vi "Client.vi"() -> ()   [LabVIEW 2023]
uses:
  <vilib>/Utility/error.llb/Trim Whitespace One-Sided.vi
  System.Speech
  <vilib>/Utility/file.llb/Read Delimited Spreadsheet (string).vi
  System.Windows.Forms
panel:
  in  "Path":path
  out "Boolean 2":bool
  in  "password 3":string
  in  "Username 2":string
  out "element":string
  out "String":string
  out "Boolean":bool
  out "CorrectPassword":string[](array[string])
  out "Username":string[](array[string])
  out "Numeric":dbl
  out "keep actual volume":dbl
  in  "WindowsMediaPlayer":refnum<k7>(container)
  in  "Tab Control":T1(tab)
  in  "log Button":bool
  out "Gauge":dbl(knob) scale=0.0..260.0
  in  "Welcome Back button":bool
  in  "login Button":bool
  in  "back to welcome back":bool
  out "current time":timestamp format="%<%x>T"
  out "current time 2":timestamp format="%<%I:%M %p>T"
  in  "Password 2":T2
  out "Password":string
  in  "Outer Control":bool
  in  "Inner Control":bool
  in  "Main Menu Log Out":bool
  in  "Radio":bool
  in  "Broswer":bool
  in  "Door Control":bool
  out "current time 22":timestamp format="%<%x>T"
  out "current time 21":timestamp format="%<%I:%M %p>T"
  in  "Door control Back to Main Menu":bool
  in  "Back Left Door":bool
  in  "Back Right Door":bool
  in  "Front Right Door":bool
  in  "Close All Doors":bool
  in  "Lock All Doors":bool
  in  "Front Left Door":bool
  out "current time 4":timestamp format="%<%x>T"
  out "current time 3":timestamp format="%<%I:%M %p>T"
  in  "Window  Child Lock":bool
  in  "Close All Windows":bool
  in  "Close Moonroof":bool
  in  "Trunk 2":bool
  in  "Bonnet 2":bool
  in  "Right Back Window":dbl(knob) scale=0.0..100.0
  in  "Right Front Window":dbl(knob) scale=0.0..100.0
  in  "Left Back Window":dbl(knob) scale=0.0..100.0
  in  "Left Front Window":dbl(knob) scale=0.0..100.0
  in  "Outer Control Back to Main Menu":bool
  in  "High Light Beam":bool
  in  "Low Light Beam":bool
  out "current time 6":timestamp format="%<%x>T"
  out "current time 5":timestamp format="%<%I:%M %p>T"
  in  "Oil Tank":bool
  in  "Siri button":bool
  in  "View 360":bool
  in  "Tempurature":u8(slide) scale=16.0..24.0
  out "Numeric 2":dbl
  out "Ac light":bool
  in  "On/Off Ac":bool
  in  "On/Off fan":bool
  out "Numeric 3":dbl
  in  "Call":bool
  in  "Password 4":T3
  out "Password 3":string
  in  "Inner Control Back to Main Menu":bool
  out "fan light":bool
  in  "Fan Speed":u8(slide) scale=1.0..5.0
  in  "Double Signal":bool
  out "current time 24":timestamp format="%<%x>T"
  out "current time 23":timestamp format="%<%I:%M %p>T"
  out "Display channel":string
  in  "ONOFF":bool
  in  "Radio Back to main menu":bool
  in  "Unmute":bool
  in  "109.90":bool
  in  "98.80":bool
  in  "105.90":bool
  in  "92.90":bool
  in  "102.90":bool
  in  "91.10":bool
  in  "101.90":bool
  in  "89.90":bool
  in  "Volume slider":u8(slide) scale=0.0..100.0
  out "current time 10":timestamp format="%<%x>T"
  out "current time 9":timestamp format="%<%I:%M %p>T"
  in  "Miscrsoft button":bool
  in  "Netflix Button":bool
  in  "Enter Url":string
  in  "Browser Back to Main Menu":bool
  in  "Gmail button":bool
  in  "Facebook button":bool
  out "current time 8":timestamp format="%<%x>T"
  out "current time 7":timestamp format="%<%I:%M %p>T"
  in  "Search Button":bool
  in  "Google Button":bool
  in  "Display Browser Back to main menu":bool
  out "current time 12":timestamp format="%<%x>T"
  out "current time 11":timestamp format="%<%I:%M %p>T"
  in  "WebBrowser":refnum<k24>(container)
  in  "360view back to main menu":bool
  out "current time 16":timestamp format="%<%x>T"
  out "current time 15":timestamp format="%<%I:%M %p>T"
  # "Welcome Back"
  # "PROTON AZ5"
  # "Enter Passcode"
  # "Main Menu"
  # "Door\nControl"
  # "Outer \nControl"
  # "Phone Call"
  # "Inner \nControl"
  # "Radio"
  # "Browser"
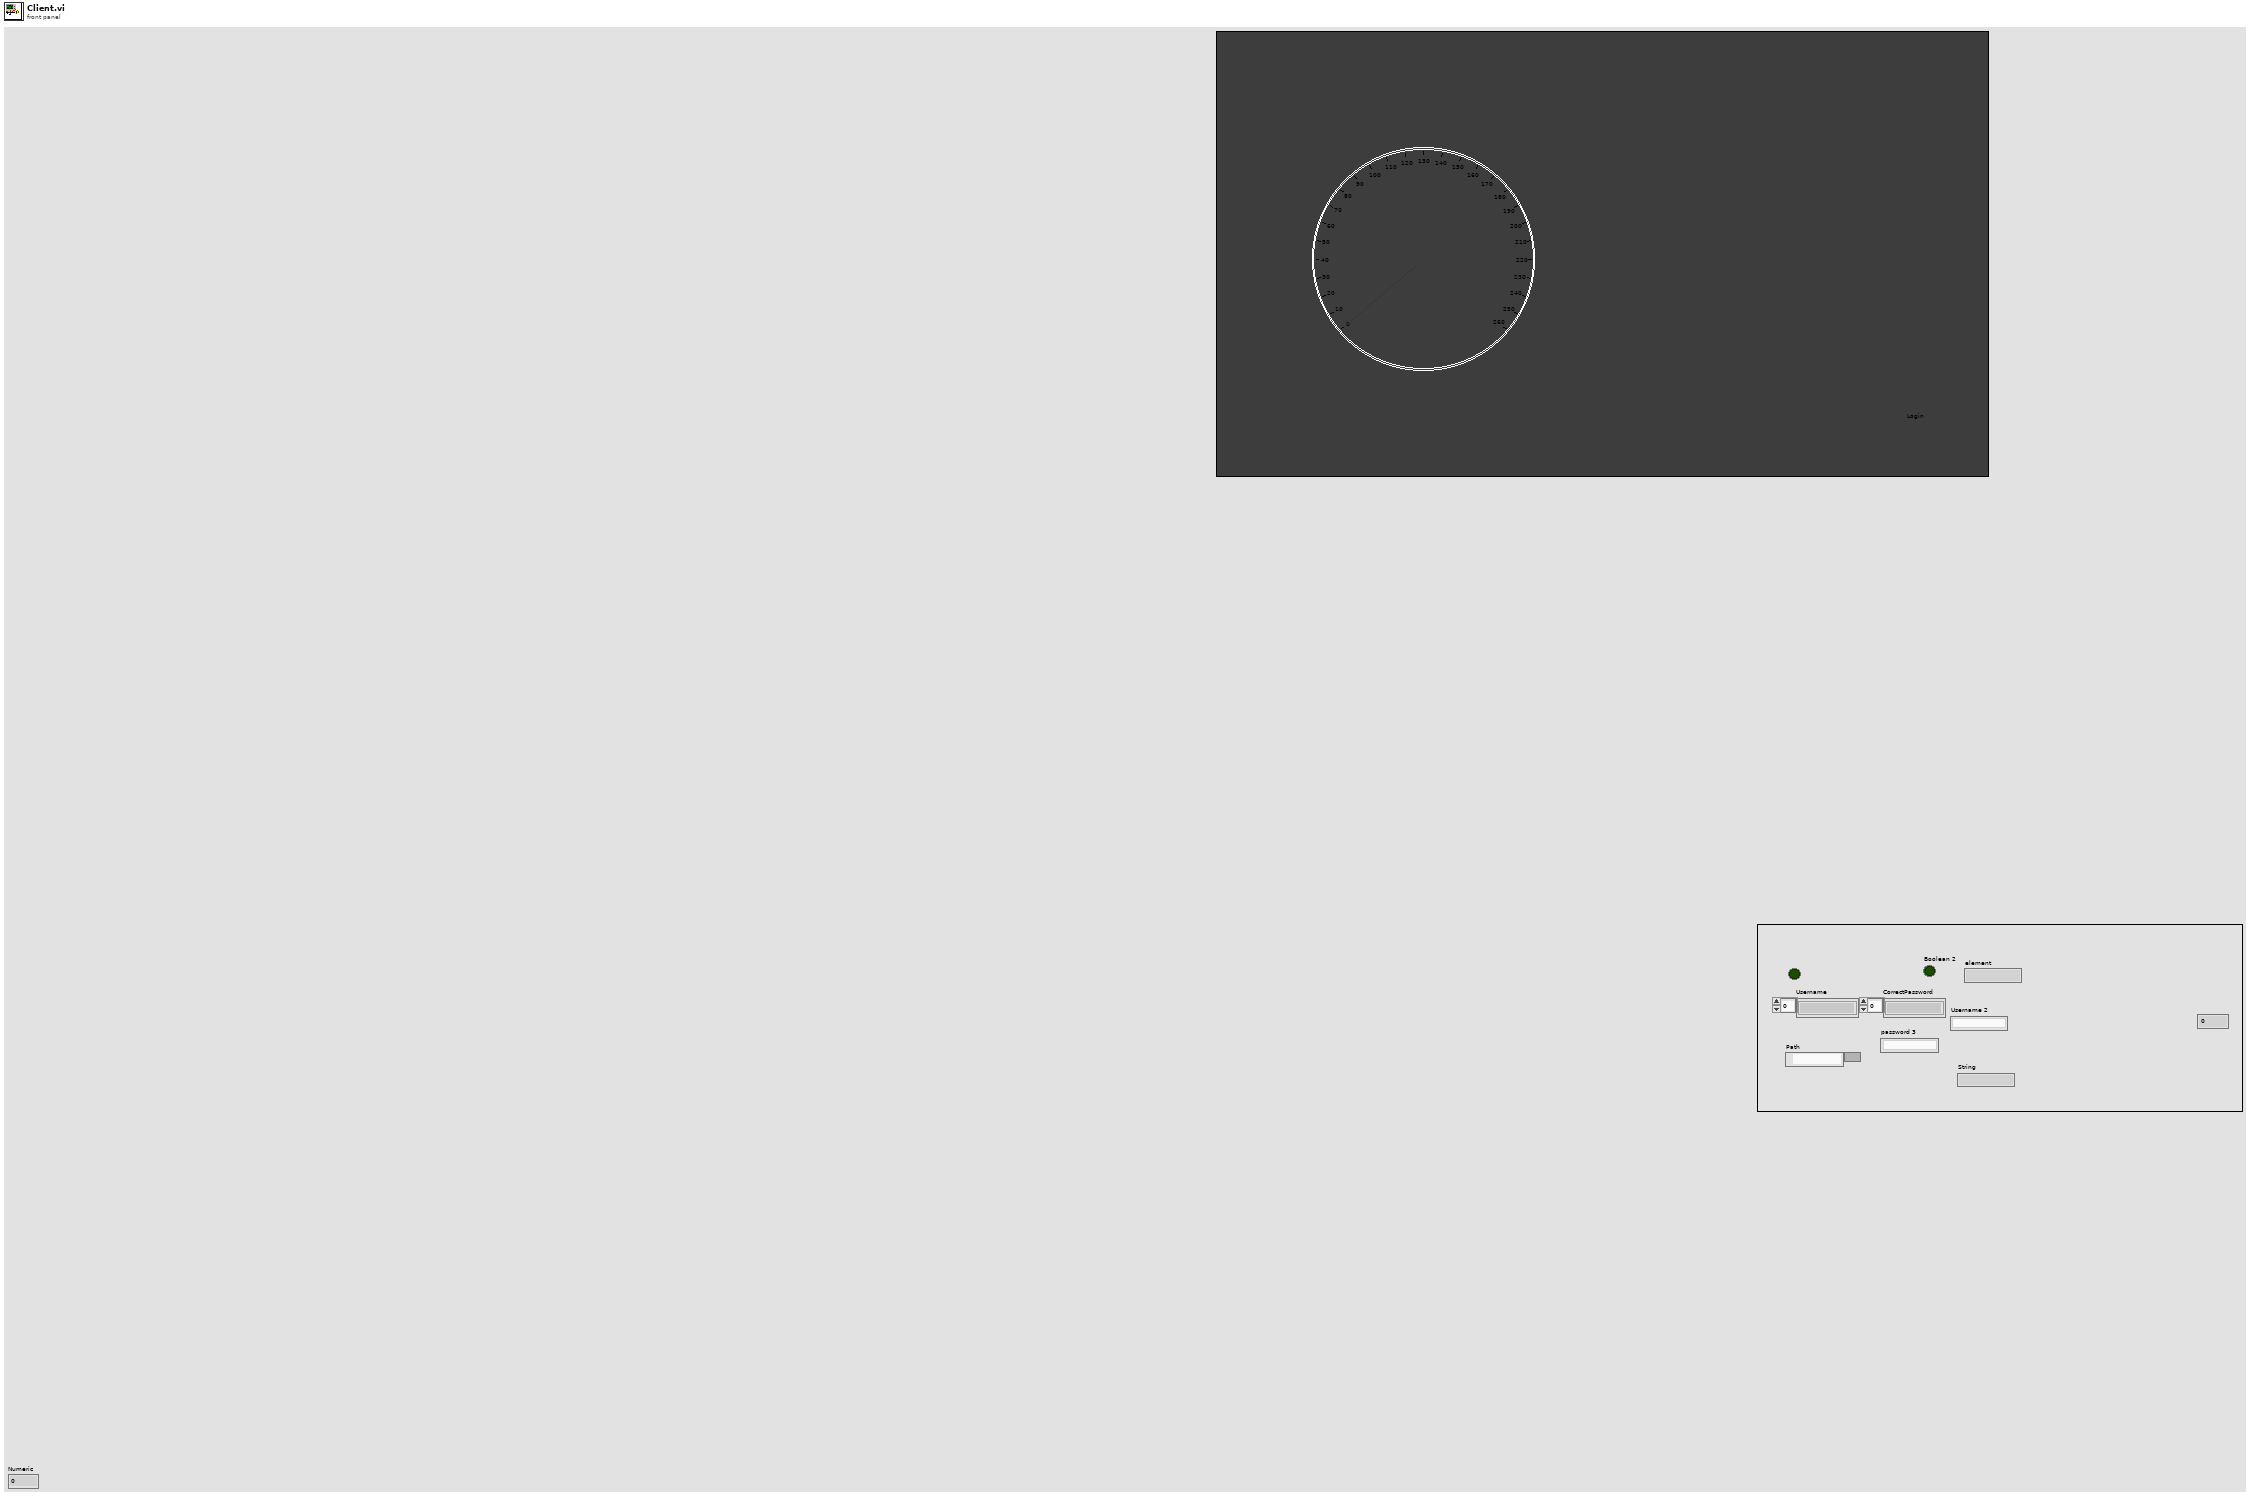
[diagram p1: front panel]
types:
  T1 = enum32{"Meter", "Login Page", "Main Menu", "Door Control", "Outer Control", "Inner Control", "Radio", "Browser", "Display Browser", "360view"}
  T2 = cluster{"1":bool, "2":bool, "4":bool, "5":bool, "6":bool, "7":bool, "8":bool, "9":bool, "0":bool, "3":bool, "Refresh Button":bool}
  T3 = cluster{"Call N1":bool, "Call N2":bool, "Call N3":bool, "Call N4":bool, "Call N5":bool, "Call N6":bool, "Call N7":bool, "Call N8":bool, "Call N9":bool, "Call N0":bool, "Clear":bool}
  T4 = enum32{"Login Page", "Menu Page", "Door Page", "Light Page", "Window Page", "Radio Page", "Browsing Page", "Advanced Setting", "Profile Page"}
  T5 = enum8{"Enabled", "Disabled", "Disabled and Grayed Out"}
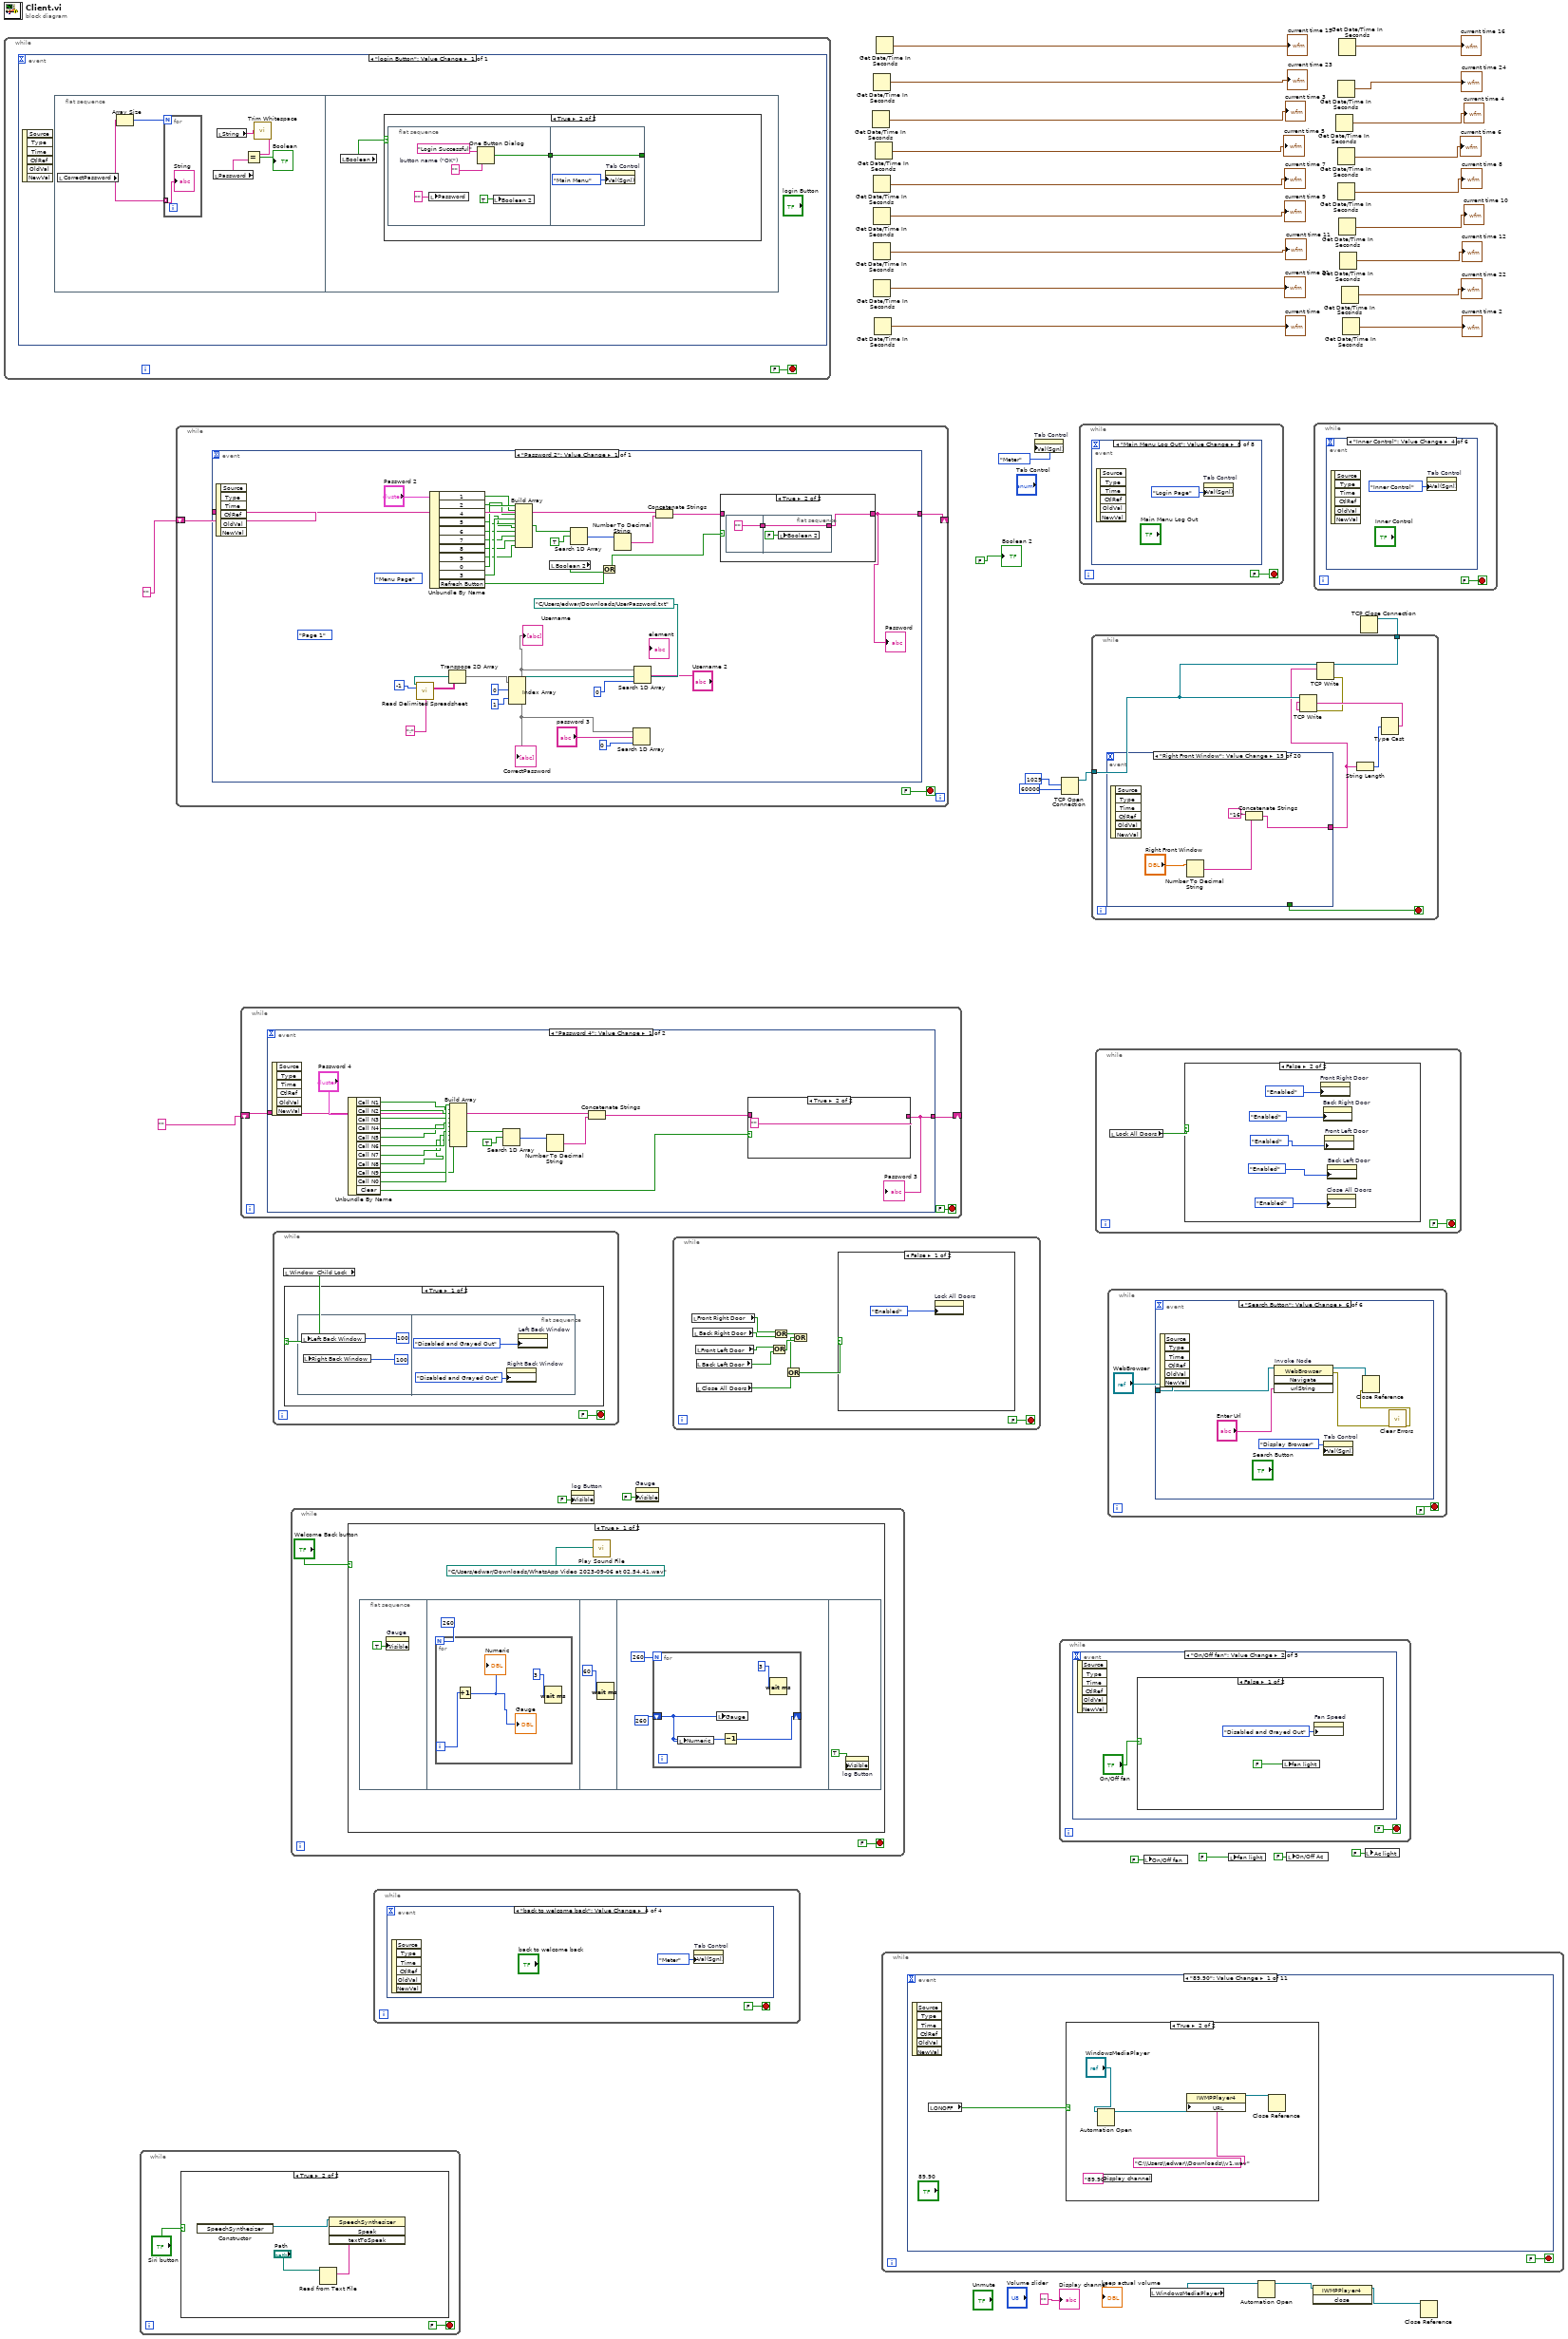
[diagram p0: block diagram]
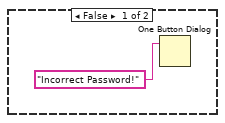
[diagram p3: hidden frame]
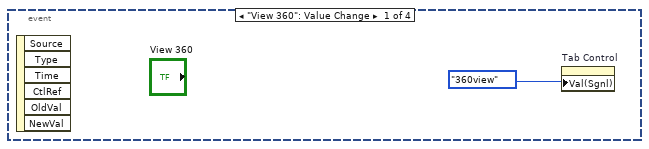
[diagram p4: hidden frame]
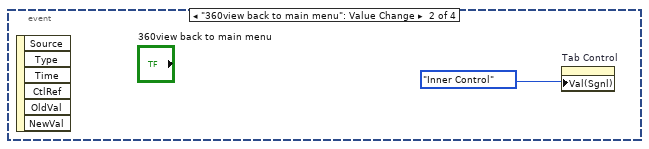
[diagram p5: hidden frame]
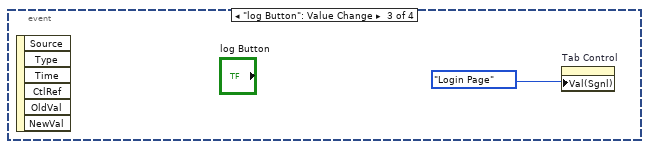
[diagram p6: hidden frame]
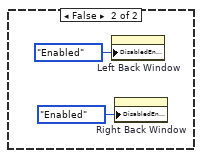
[diagram p8: hidden frame]
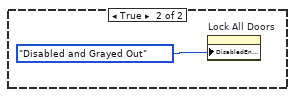
[diagram p9: hidden frame]
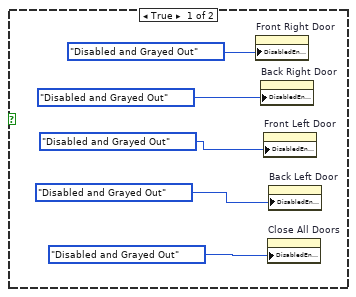
[diagram p10: hidden frame]
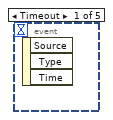
[diagram p11: hidden frame]
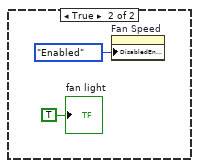
[diagram p12: hidden frame]
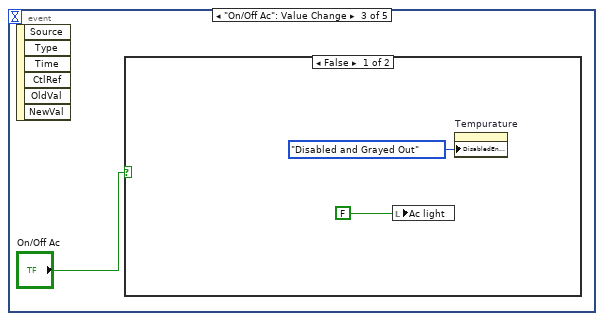
[diagram p13: hidden frame]
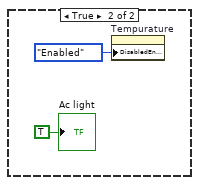
[diagram p14: hidden frame]
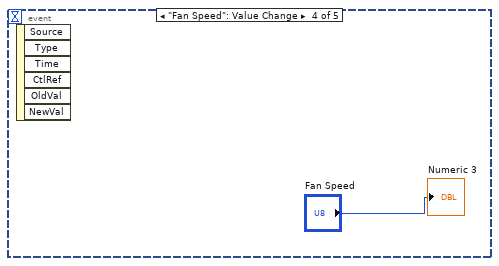
[diagram p15: hidden frame]
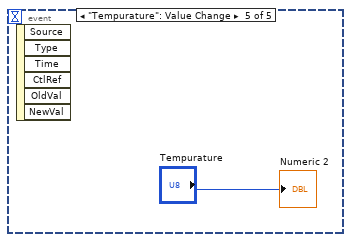
[diagram p16: hidden frame]
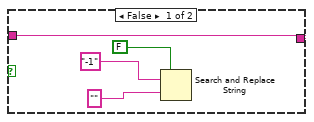
[diagram p17: hidden frame]
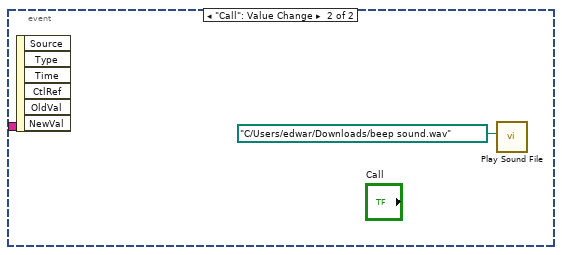
[diagram p18: hidden frame]
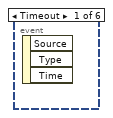
[diagram p19: hidden frame]
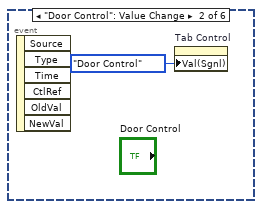
[diagram p20: hidden frame]
diagram:
  n1 = while {
    stop <- FALSE stop-if-true
    n2 = event shown="[0] \"login Button\": Value Change" {
      selector: _ -> [_]
      dyn-events: _ -> [_]
      timeout: _ -> [_]
      event "login Button": Value Change {
        n3 = event-data() -> ()  [unwired: 1 in, 6 out]
        n4 = flat-sequence {
          frame #0 {
            n5 = local read "CorrectPassword"() -> (w42:string[])
            n6 = Array Size(array=w42) -> (size(s)=w43:i32)
            n7 = for {
              N: w43 -> [_]
              tunnel: w42 -> [w44] mode=indexing
              "String" <- w44
            }
            n8 = local read "Password"() -> (w38:string)
            n9 = local read "String"() -> (w40:string)
            n10 = call <vilib>:"Trim Whitespace.vi"("string"=w40) -> ("trimmed string"=w39:string)  [unwired: 1 in]
            n11 = Equal?(x=w39, y=w38) -> (x = y?=→"Boolean":bool)
          }
          frame #1 {
            n12 = local read "Boolean"() -> (w45:bool)
            n13 = case shown="True" w45 {
              frame False {
                n14 = One Button Dialog(message="Incorrect Password!") -> ()  [unwired: 1 in, 1 out]
              }
              frame True {
                n15 = flat-sequence {
                  tunnel: [w48] -> w47
                  tunnel: [w53] -> _
                  tunnel: w47 -> [w53]
                  frame #0 {
                    w51 = ""  # button name ("OK")
                    n16 = local write "Password"("" ("Passsword")) -> ()
                    n17 = One Button Dialog(message="Login Successful", button name ("OK")=w51) -> (true=w48:bool)
                    n18 = local write "Boolean 2"(TRUE ("Boolean 2")) -> ()
                  }
                  frame #1 {
                    n19 = property on="Tab Control" class="TabCtl (strict)"("Val(Sgnl)"=T1."Main Menu" ("Value (Signaling)")) -> ()  [unwired: 2 in, 2 out]
                  }
                }
              }
            }
          }
        }
      }
    }
  }
  n20 = while {
    stop <- FALSE stop-if-true
    n21 = case shown="True" "Siri button" {
      frame False {
      }
      frame True {
        n22 = constructor class="SpeechSynthesizer"() -> (reference out=w59:refnum<k24>)  [unwired: 3 in, 2 out]
        n23 = Read from Text File(file (use dialog)="Path") -> (text=w57:string)  [unwired: 3 in, 3 out]
        n24 = invoke class="SpeechSynthesizer" method="Speak"(reference=w59, "textToSpeak"=w57) -> ()  [unwired: 2 in, 4 out]
      }
    }
  }
  n25 = while {
    shift-right: [w60] -> _
    shift-left: "" -> [w61]
    stop <- FALSE stop-if-true
    n26 = event shown="[0] \"Password 2\": Value Change" {
      selector: _ -> [_]
      dyn-events: _ -> [_]
      timeout: _ -> [_]
      tunnel: w61 -> [w92]
      tunnel: [w68] -> w60
      event "Password 2": Value Change {
        (unwired) T4."Menu Page" ("Value (Signaling)")
        (unwired) enum32{"Page 1", "Page 2"}."Page 1" ("Tab Control 12")
        n27 = event-data() -> ()  [unwired: 1 in, 6 out]
        n28 = call-poly <vilib>:"Read Delimited Spreadsheet.vi"("file path (dialog if empty)"=path "C:/Users/edwar/Downloads/UserPassword.txt", "number of rows (all:-1)"=-1, "delimiter (\\t)"=":" ("delimiter (\\t)")) -> ("all rows"=w79:string[][])  [unwired: 7 in, 5 out]
        n29 = Unbundle By Name "Unbundle By Name"("Password 2") -> ("1"=w90:bool, "2"=w89:bool, "4"=w87:bool, "5"=w86:bool, "6"=w85:bool, "7"=w84:bool, "8"=w83:bool, "9"=w82:bool, "0"=w91:bool, "3"=w88:bool, "Refresh Button"=w65:bool)
        n30 = Transpose 2D Array(2D array=w79) -> (transposed array=w78:string[][])
        n31 = Index Array(array=w78, index (row) #1=0 ("index (row)"), index (row) #2=1 ("index (row)")) -> (element #1=w70:string[], element #2=w69:string[])  [unwired: 2 in]
        "Username" <- w70
        "CorrectPassword" <- w69
        n32 = Build Array "Build Array"(w91, w90, w89, w88, w87, w86, w85, w84, w83, w82) -> (w95:bool[])
        n33 = local read "Boolean 2"() -> (w63:bool)
        n34 = Search 1D Array(1D array=w95, element=TRUE) -> (index of element=w94:i32)  [unwired: 1 in]
        n35 = Or(x=w65, y=w63) -> (x .or. y?=w64:bool)
        n36 = Number To Decimal String(number=w94) -> (decimal integer string=w93:string)  [unwired: 1 in]
        n37 = Search 1D Array(1D array=w69, element="password 3", start index (0)=0) -> ()  [unwired: 1 out]
        n38 = Search 1D Array(1D array=w70, element="Username 2", start index (0)=0) -> ()  [unwired: 1 out]
        n39 = Concatenate Strings "Concatenate Strings"(w92, w93) -> (w80:string)
        n40 = case shown="True" w64 {
          tunnel: w80 -> [w97 _]
          tunnel: [w97 w102] -> w68
          frame False {
            n41 = Search and Replace String(replace all?=FALSE ("replace all? (F)"), input string="", search string="-1") -> ()  [unwired: 5 in, 4 out]
          }
          frame True {
            n42 = flat-sequence {
              tunnel: [""] -> w101
              tunnel: [w105] -> w102
              tunnel: w101 -> [w105]
              frame #0 {
              }
              frame #1 {
                n43 = local write "Boolean 2"(FALSE ("Boolean 2")) -> ()
              }
            }
          }
        }
        "Password" <- w68
      }
    }
  }
  n44 = while {
    shift-right: [w108] -> _
    shift-left: "" -> [w107]
    stop <- FALSE stop-if-true
    n45 = event shown="[0] \"Password 4\": Value Change" {
      selector: _ -> [_ _]
      dyn-events: _ -> [_ _]
      timeout: _ -> [_ _]
      tunnel: [w110 _] -> w108
      tunnel: w107 -> [w111 _]
      event "Password 4": Value Change {
        n46 = event-data() -> ()  [unwired: 1 in, 6 out]
        n47 = Unbundle By Name("Password 4") -> ("Call N1"=w125:bool, "Call N2"=w124:bool, "Call N3"=w123:bool, "Call N4"=w122:bool, "Call N5"=w121:bool, "Call N6"=w120:bool, "Call N7"=w119:bool, "Call N8"=w118:bool, "Call N9"=w117:bool, "Call N0"=w126:bool, "Clear"=w109:bool)
        n48 = Build Array "Build Array"(w126, w125, w124, w123, w122, w121, w120, w119, w118, w117) -> (w112:bool[])
        n49 = Search 1D Array(1D array=w112, element=TRUE) -> (index of element=w116:i32)  [unwired: 1 in]
        n50 = Number To Decimal String(number=w116) -> (decimal integer string=w115:string)  [unwired: 1 in]
        n51 = Concatenate Strings "Concatenate Strings"(w111, w115) -> (w113:string)
        n52 = case shown="True" w109 {
          tunnel: w113 -> [w128 _]
          tunnel: [w128 ""] -> w110
          frame False {
            n53 = Search and Replace String(replace all?=FALSE ("replace all? (F)"), input string="", search string="-1") -> ()  [unwired: 5 in, 4 out]
          }
          frame True {
          }
        }
        "Password 3" <- w110
      }
      event "Call": Value Change {
        n54 = event-data() -> ()  [unwired: 1 in, 6 out]
        n55 = call <vilib>:"Play Sound File.vi"("path"=path "C:/Users/edwar/Downloads/beep sound.wav") -> ()  [unwired: 9 in, 2 out]
      }
    }
  }
  n56 = while {
    stop <- FALSE stop-if-true
    n57 = local read "Window  Child Lock"() -> (w134:bool)
    n58 = case shown="True" w134 {
      frame True {
        n59 = flat-sequence {
          frame #0 {
            n60 = local write "Left Back Window"(100) -> ()
            n61 = local write "Right Back Window"(100) -> ()
          }
          frame #1 {
            n62 = property on="Right Back Window" class="Knob (strict)"("DisabledEnum"=T5."Disabled and Grayed Out" ("Disabled")) -> ()  [unwired: 2 in, 2 out]
            n63 = property on="Left Back Window" class="Knob (strict)"("DisabledEnum"=T5."Disabled and Grayed Out" ("Disabled")) -> ()  [unwired: 2 in, 2 out]
          }
        }
      }
      frame False {
        n64 = property on="Left Back Window" class="Knob (strict)"("DisabledEnum"=T5."Enabled" ("Disabled")) -> ()  [unwired: 2 in, 2 out]
        n65 = property on="Right Back Window" class="Knob (strict)"("DisabledEnum"=T5."Enabled" ("Disabled")) -> ()  [unwired: 2 in, 2 out]
      }
    }
  }
  n66 = while {
    stop <- FALSE stop-if-true
    n67 = case shown="True" "Welcome Back button" {
      frame True {
        n68 = flat-sequence {
          frame #0 {
            n69 = property on="Gauge" class="Knob (strict)"("Visible"=TRUE) -> ()  [unwired: 2 in, 2 out]
          }
          frame #1 {
            n70 = for {
              N: 260 -> [_]
              i -> [w149]
              n71 = Increment(x=w149) -> (x+1=→"Numeric" →"Gauge":i32)
              n72 = Wait (ms)(milliseconds to wait=u32 3) -> ()  [unwired: 1 out]
            }
          }
          frame #2 {
            n73 = Wait (ms)(milliseconds to wait=u32 60) -> ()  [unwired: 1 out]
          }
          frame #3 {
            n74 = for {
              N: 260 -> [_]
              shift-right: [w153] -> _
              shift-left: 260 -> [w154]
              n75 = local write "Numeric"(w154) -> ()
              n76 = local write "Gauge"(w154) -> ()
              n77 = Decrement(x=w154) -> (x-1=w153:i32)
              n78 = Wait (ms)(milliseconds to wait=u32 3) -> ()  [unwired: 1 out]
            }
          }
          frame #4 {
            n79 = property on="log Button" class="Bool"("Visible"=TRUE) -> ()  [unwired: 2 in, 2 out]
          }
        }
        n80 = call <vilib>:"Play Sound File.vi"("path"=path "C:/Users/edwar/Downloads/WhatsApp Video 2023-09-06 at 02.54.41.wav") -> ()  [unwired: 9 in, 2 out]
      }
      frame False {
      }
    }
  }
  n81 = while {
    stop <- FALSE stop-if-true
    n82 = event shown="[3] \"back to welcome back\": Value Change" {
      selector: _ -> [_ _ _ _]
      dyn-events: _ -> [_ _ _ _]
      timeout: _ -> [_ _ _ _]
      event "View 360": Value Change {
        n83 = event-data() -> ()  [unwired: 1 in, 6 out]
        n84 = property on="Tab Control" class="TabCtl (strict)"("Val(Sgnl)"=T1."360view" ("Value (Signaling)")) -> ()  [unwired: 2 in, 2 out]
      }
      event "360view back to main menu": Value Change {
        n85 = event-data() -> ()  [unwired: 1 in, 6 out]
        n86 = property on="Tab Control" class="TabCtl (strict)"("Val(Sgnl)"=T1."Inner Control" ("Value (Signaling)")) -> ()  [unwired: 2 in, 2 out]
      }
      event "log Button": Value Change {
        n87 = event-data() -> ()  [unwired: 1 in, 6 out]
        n88 = property on="Tab Control" class="TabCtl (strict)"("Val(Sgnl)"=T1."Login Page" ("Value (Signaling)")) -> ()  [unwired: 2 in, 2 out]
      }
      event "back to welcome back": Value Change {
        n89 = event-data() -> ()  [unwired: 1 in, 6 out]
        n90 = property on="Tab Control" class="TabCtl (strict)"("Val(Sgnl)"=T1."Meter" ("Value (Signaling)")) -> ()  [unwired: 2 in, 2 out]
      }
    }
  }
  n91 = property on="log Button" class="Bool"("Visible"=FALSE) -> ()  [unwired: 2 in, 2 out]
  n92 = property on="Gauge" class="Knob (strict)"("Visible"=FALSE) -> ()  [unwired: 2 in, 2 out]
  n93 = while {
    stop <- FALSE stop-if-true
    n94 = local read "Front Right Door"() -> (w171:bool)
    n95 = local read "Back Right Door"() -> (w168:bool)
    n96 = local read "Front Left Door"() -> (w167:bool)
    n97 = local read "Back Left Door"() -> (w166:bool)
    n98 = local read "Close All Doors"() -> (w164:bool)
    n99 = Or(x=w167, y=w166) -> (x .or. y?=w169:bool)
    n100 = Or(x=w171, y=w168) -> (x .or. y?=w170:bool)
    n101 = Or(x=w170, y=w169) -> (x .or. y?=w163:bool)
    n102 = Or(x=w163, y=w164) -> (x .or. y?=w162:bool)
    n103 = case shown="False" w162 {
      frame False {
        n104 = property on="Lock All Doors" class="Bool (strict)"("DisabledEnum"=T5."Enabled" ("Disabled")) -> ()  [unwired: 2 in, 2 out]
      }
      frame True {
        n105 = property on="Lock All Doors" class="Bool (strict)"("DisabledEnum"=T5."Disabled and Grayed Out" ("Disabled")) -> ()  [unwired: 2 in, 2 out]
      }
    }
  }
  n106 = Get Date/Time In Seconds() -> (seconds since 1Jan1904=→"current time 3":timestamp)
  n107 = Get Date/Time In Seconds() -> (seconds since 1Jan1904=→"current time 7":timestamp)
  n108 = Get Date/Time In Seconds() -> (seconds since 1Jan1904=→"current time 9":timestamp)
  n109 = Get Date/Time In Seconds() -> (seconds since 1Jan1904=→"current time 11":timestamp)
  n110 = Get Date/Time In Seconds() -> (seconds since 1Jan1904=→"current time 23":timestamp)
  n111 = Get Date/Time In Seconds() -> (seconds since 1Jan1904=→"current time 21":timestamp)
  n112 = Get Date/Time In Seconds() -> (seconds since 1Jan1904=→"current time":timestamp)
  n113 = Get Date/Time In Seconds() -> (seconds since 1Jan1904=→"current time 5":timestamp)
  n114 = Get Date/Time In Seconds() -> (seconds since 1Jan1904=→"current time 15":timestamp)
  n115 = while {
    stop <- FALSE stop-if-true
    n116 = event shown="[0] \"89.90\": Value Change" {
      selector: _ -> [_ _ _ _ _ _ _ _ _ _ _]
      dyn-events: _ -> [_ _ _ _ _ _ _ _ _ _ _]
      timeout: _ -> [_ _ _ _ _ _ _ _ _ _ _]
      event "89.90": Value Change {
        n117 = event-data() -> ()  [unwired: 1 in, 6 out]
        n118 = local read "ONOFF"() -> (w175:bool)
        n119 = case shown="True" w175 {
          frame False {
            n120 = One Button Dialog(message="Please turn on the radio", button name ("OK")="") -> ()  [unwired: 1 out]
          }
          frame True {
            n121 = local write "Display channel"("89.90" ("String")) -> ()
            n122 = Automation Open(Automation Refnum="WindowsMediaPlayer") -> (Automation Refnum=w180:refnum<k7>)  [unwired: 3 in, 1 out]
            n123 = property class="IWMPPlayer4"(reference=w180, "URL"="C:\\Users\\edwar\\Downloads\\v1.wav") -> (reference out=w182:refnum<k7>)  [unwired: 1 in, 1 out]
            n124 = Close Reference(reference=w182) -> ()  [unwired: 1 in, 1 out]
          }
        }
      }
      event "91.10": Value Change {
        n125 = event-data() -> ()  [unwired: 1 in, 6 out]
        n126 = local read "ONOFF"() -> (w183:bool)
        n127 = case shown="True" w183 {
          frame False {
            n128 = One Button Dialog(message="Please turn on the radio", button name ("OK")="") -> ()  [unwired: 1 out]
          }
          frame True {
            n129 = local read "WindowsMediaPlayer"() -> (w186:refnum<k7>)
            n130 = local write "Display channel"("91.90" ("String")) -> ()
            n131 = Automation Open(Automation Refnum=w186) -> (Automation Refnum=w189:refnum<k7>)  [unwired: 3 in, 1 out]
            n132 = property class="IWMPPlayer4"(reference=w189, "URL"="C:\\Users\\edwar\\Downloads\\v2.wav") -> (reference out=w190:refnum<k7>)  [unwired: 1 in, 1 out]
            n133 = Close Reference(reference=w190) -> ()  [unwired: 1 in, 1 out]
          }
        }
      }
      event "92.90": Value Change {
        n134 = event-data() -> ()  [unwired: 1 in, 6 out]
        n135 = local read "ONOFF"() -> (w191:bool)
        n136 = case shown="True" w191 {
          frame False {
            n137 = One Button Dialog(message="Please turn on the radio", button name ("OK")="") -> ()  [unwired: 1 out]
          }
          frame True {
            n138 = local read "WindowsMediaPlayer"() -> (w194:refnum<k7>)
            n139 = local write "Display channel"("92.90" ("String")) -> ()
            n140 = Automation Open(Automation Refnum=w194) -> (Automation Refnum=w197:refnum<k7>)  [unwired: 3 in, 1 out]
            n141 = property class="IWMPPlayer4"(reference=w197, "URL"="C:\\Users\\edwar\\Downloads\\v3.wav") -> (reference out=w198:refnum<k7>)  [unwired: 1 in, 1 out]
            n142 = Close Reference(reference=w198) -> ()  [unwired: 1 in, 1 out]
          }
        }
      }
      event "98.80": Value Change {
        n143 = event-data() -> ()  [unwired: 1 in, 6 out]
        n144 = local read "ONOFF"() -> (w199:bool)
        n145 = case shown="True" w199 {
          frame False {
            n146 = One Button Dialog(message="Please turn on the radio", button name ("OK")="") -> ()  [unwired: 1 out]
          }
          frame True {
            n147 = local read "WindowsMediaPlayer"() -> (w202:refnum<k7>)
            n148 = local write "Display channel"("98.80" ("String")) -> ()
            n149 = Automation Open(Automation Refnum=w202) -> (Automation Refnum=w205:refnum<k7>)  [unwired: 3 in, 1 out]
            n150 = property class="IWMPPlayer4"(reference=w205, "URL"="C:\\Users\\edwar\\Downloads\\v4.wav") -> (reference out=w206:refnum<k7>)  [unwired: 1 in, 1 out]
            n151 = Close Reference(reference=w206) -> ()  [unwired: 1 in, 1 out]
          }
        }
      }
      event "101.90": Value Change {
        n152 = event-data() -> ()  [unwired: 1 in, 6 out]
        n153 = local read "ONOFF"() -> (w207:bool)
        n154 = case shown="True" w207 {
          frame False {
            n155 = One Button Dialog(message="Please turn on the radio", button name ("OK")="") -> ()  [unwired: 1 out]
          }
          frame True {
            n156 = local read "WindowsMediaPlayer"() -> (w210:refnum<k7>)
            n157 = local write "Display channel"("101.90" ("String")) -> ()
            n158 = Automation Open(Automation Refnum=w210) -> (Automation Refnum=w213:refnum<k7>)  [unwired: 3 in, 1 out]
            n159 = property class="IWMPPlayer4"(reference=w213, "URL"="C:\\Users\\edwar\\Downloads\\v5.wav") -> (reference out=w214:refnum<k7>)  [unwired: 1 in, 1 out]
            n160 = Close Reference(reference=w214) -> ()  [unwired: 1 in, 1 out]
          }
        }
      }
      event "102.90": Value Change {
        n161 = event-data() -> ()  [unwired: 1 in, 6 out]
        n162 = local read "ONOFF"() -> (w215:bool)
        n163 = case shown="True" w215 {
          frame False {
            n164 = One Button Dialog(message="Please turn on the radio", button name ("OK")="") -> ()  [unwired: 1 out]
          }
          frame True {
            n165 = local read "WindowsMediaPlayer"() -> (w218:refnum<k7>)
            n166 = local write "Display channel"("102.90" ("String")) -> ()
            n167 = Automation Open(Automation Refnum=w218) -> (Automation Refnum=w221:refnum<k7>)  [unwired: 3 in, 1 out]
            n168 = property class="IWMPPlayer4"(reference=w221, "URL"="C:\\Users\\edwar\\Downloads\\v6.wav") -> (reference out=w222:refnum<k7>)  [unwired: 1 in, 1 out]
            n169 = Close Reference(reference=w222) -> ()  [unwired: 1 in, 1 out]
          }
        }
      }
      event "105.90": Value Change {
        n170 = event-data() -> ()  [unwired: 1 in, 6 out]
        n171 = local read "ONOFF"() -> (w223:bool)
        n172 = case shown="True" w223 {
          frame False {
            n173 = One Button Dialog(message="Please turn on the radio", button name ("OK")="") -> ()  [unwired: 1 out]
          }
          frame True {
            n174 = local read "WindowsMediaPlayer"() -> (w226:refnum<k7>)
            n175 = local write "Display channel"("105.90" ("String")) -> ()
            n176 = Automation Open(Automation Refnum=w226) -> (Automation Refnum=w229:refnum<k7>)  [unwired: 3 in, 1 out]
            n177 = property class="IWMPPlayer4"(reference=w229, "URL"="C:\\Users\\edwar\\Downloads\\v7.wav") -> (reference out=w230:refnum<k7>)  [unwired: 1 in, 1 out]
            n178 = Close Reference(reference=w230) -> ()  [unwired: 1 in, 1 out]
          }
        }
      }
      event "109.90": Value Change {
        n179 = event-data() -> ()  [unwired: 1 in, 6 out]
        n180 = local read "ONOFF"() -> (w231:bool)
        n181 = case shown="True" w231 {
          frame False {
            n182 = One Button Dialog(message="Please turn on the radio", button name ("OK")="") -> ()  [unwired: 1 out]
          }
          frame True {
            n183 = local read "WindowsMediaPlayer"() -> (w234:refnum<k7>)
            n184 = local write "Display channel"("109.90" ("String")) -> ()
            n185 = Automation Open(Automation Refnum=w234) -> (Automation Refnum=w237:refnum<k7>)  [unwired: 3 in, 1 out]
            n186 = property class="IWMPPlayer4"(reference=w237, "URL"="C:\\Users\\edwar\\Downloads\\v8.wav") -> (reference out=w238:refnum<k7>)  [unwired: 1 in, 1 out]
            n187 = Close Reference(reference=w238) -> ()  [unwired: 1 in, 1 out]
          }
        }
      }
      event "Unmute": Value Change {
        n188 = event-data() -> ()  [unwired: 1 in, 6 out]
        n189 = local read "Unmute"() -> (w239:bool)
        n190 = case shown="True" w239 {
          frame True {
            n191 = flat-sequence {
              frame #0 {
                n192 = local read "Volume slider"() -> (w240:u8)
                n193 = local write "keep actual volume"(w240) -> ()
              }
              frame #1 {
                n194 = local write "Volume slider"(u8 0 ("Volume slider")) -> ()
              }
              frame #2 {
                n195 = local read "WindowsMediaPlayer"() -> (w246:refnum<k7>)
                n196 = Automation Open(Automation Refnum=w246) -> (Automation Refnum=w245:refnum<k7>)  [unwired: 3 in, 1 out]
                n197 = property class="IWMPPlayer4"(reference=w245) -> ("settings"=w243:refnum<k7>)  [unwired: 1 in, 2 out]
                n198 = local read "Volume slider"() -> (w242:u8)
                n199 = property class="IWMPSettings"(reference=w243, "volume"=w242) -> (reference out=w244:refnum<k7>)  [unwired: 1 in, 1 out]
                n200 = Close Reference(reference=w244) -> ()  [unwired: 1 in, 1 out]
              }
            }
          }
          frame False {
            n201 = flat-sequence {
              frame #0 {
                n202 = local read "keep actual volume"() -> (w247:dbl)
                n203 = local write "Volume slider"(w247) -> ()
              }
              frame #1 {
                n204 = local read "WindowsMediaPlayer"() -> (w251:refnum<k7>)
                n205 = Automation Open(Automation Refnum=w251) -> (Automation Refnum=w250:refnum<k7>)  [unwired: 3 in, 1 out]
                n206 = property class="IWMPPlayer4"(reference=w250) -> ("settings"=w248:refnum<k7>)  [unwired: 1 in, 2 out]
                n207 = local read "Volume slider"() -> (w252:u8)
                n208 = property class="IWMPSettings"(reference=w248, "volume"=w252) -> (reference out=w249:refnum<k7>)  [unwired: 1 in, 1 out]
                n209 = Close Reference(reference=w249) -> ()  [unwired: 1 in, 1 out]
              }
            }
          }
        }
      }
      event "Volume slider": Value Change {
        n210 = event-data() -> ()  [unwired: 1 in, 6 out]
        n211 = local read "WindowsMediaPlayer"() -> (w254:refnum<k7>)
        n212 = Automation Open(Automation Refnum=w254) -> (Automation Refnum=w255:refnum<k7>)  [unwired: 3 in, 1 out]
        n213 = property class="IWMPPlayer4"(reference=w255) -> ("settings"=w257:refnum<k7>)  [unwired: 1 in, 2 out]
        n214 = local read "Volume slider"() -> (w253:u8)
        n215 = property class="IWMPSettings"(reference=w257, "volume"=w253) -> (reference out=w256:refnum<k7>)  [unwired: 1 in, 1 out]
        n216 = Close Reference(reference=w256) -> ()  [unwired: 1 in, 1 out]
      }
      event "ONOFF": Value Change {
        n217 = event-data() -> ()  [unwired: 1 in, 6 out]
        n218 = case shown="True" "ONOFF" {
          frame False {
            n219 = local read "WindowsMediaPlayer"() -> (w260:refnum<k7>)
            n220 = local write "Display channel"("" ("String")) -> ()
            n221 = Automation Open(Automation Refnum=w260) -> (Automation Refnum=w261:refnum<k7>)  [unwired: 3 in, 1 out]
            n222 = property class="IWMPPlayer4"(reference=w261) -> ("controls"=w263:refnum<k7>)  [unwired: 1 in, 2 out]
            n223 = invoke class="IWMPControls" method="stop"(reference=w263) -> (reference out=w262:refnum<k7>)  [unwired: 2 in, 2 out]
            n224 = Close Reference(reference=w262) -> ()  [unwired: 1 in, 1 out]
          }
          frame True {
            n225 = local read "WindowsMediaPlayer"() -> (w265:refnum<k7>)
            n226 = Automation Open(Automation Refnum=w265) -> (Automation Refnum=w268:refnum<k7>)  [unwired: 3 in, 1 out]
            n227 = property class="IWMPPlayer4"(reference=w268) -> ("settings"=w266:refnum<k7>)  [unwired: 1 in, 2 out]
            n228 = local read "Volume slider"() -> (w264:u8)
            n229 = property class="IWMPSettings"(reference=w266, "volume"=w264) -> (reference out=w267:refnum<k7>)  [unwired: 1 in, 1 out]
            n230 = Close Reference(reference=w267) -> ()  [unwired: 1 in, 1 out]
          }
        }
      }
    }
  }
  n231 = property on="Tab Control" class="TabCtl (strict)"("Val(Sgnl)"=T1."Meter" ("Value (Signaling)")) -> ()  [unwired: 2 in, 2 out]
  n232 = while {
    stop <- FALSE stop-if-true
    n233 = event shown="[1] \"On/Off fan\": Value Change" {
      selector: _ -> [_ _ _ _ _]
      dyn-events: _ -> [_ _ _ _ _]
      timeout: _ -> [_ _ _ _ _]
      event Timeout {
        n234 = event-data() -> ()  [unwired: 1 in, 3 out]
      }
      event "On/Off fan": Value Change {
        n235 = event-data() -> ()  [unwired: 1 in, 6 out]
        n236 = case shown="False" "On/Off fan" {
          frame False {
            n237 = local write "fan light"(FALSE ("Air Conditional light")) -> ()
            n238 = property on="Fan Speed" class="Slide (strict)"("DisabledEnum"=T5."Disabled and Grayed Out" ("Disabled")) -> ()  [unwired: 2 in, 2 out]
          }
          frame True {
            n239 = property on="Fan Speed" class="Slide (strict)"("DisabledEnum"=T5."Enabled" ("Disabled")) -> ()  [unwired: 2 in, 2 out]
            "fan light" <- TRUE ("Air Conditional light")
          }
        }
      }
      event "On/Off Ac": Value Change {
        n240 = event-data() -> ()  [unwired: 1 in, 6 out]
        n241 = case shown="False" "On/Off Ac" {
          frame False {
            n242 = local write "Ac light"(FALSE ("Air Conditional light")) -> ()
            n243 = property on="Tempurature" class="Slide (strict)"("DisabledEnum"=T5."Disabled and Grayed Out" ("Disabled")) -> ()  [unwired: 2 in, 2 out]
          }
          frame True {
            n244 = property on="Tempurature" class="Slide (strict)"("DisabledEnum"=T5."Enabled" ("Disabled")) -> ()  [unwired: 2 in, 2 out]
            "Ac light" <- TRUE ("Air Conditional light")
          }
        }
      }
      event "Fan Speed": Value Change {
        n245 = event-data() -> ()  [unwired: 1 in, 6 out]
        "Numeric 3" <- "Fan Speed"
      }
      event "Tempurature": Value Change {
        n246 = event-data() -> ()  [unwired: 1 in, 6 out]
        "Numeric 2" <- "Tempurature"
      }
    }
  }
  n247 = TCP Open Connection(remote port or service name=u16 1029, timeout ms (60000)=60000) -> (connection ID=w31:refnum<k5>)  [unwired: 3 in, 1 out]
  n248 = while {
    stop <- FALSE stop-if-true
    n249 = event shown="[7] \"Main Menu Log Out\": Value Change" {
      selector: _ -> [_ _ _ _ _ _ _ _]
      dyn-events: _ -> [_ _ _ _ _ _ _ _]
      timeout: _ -> [_ _ _ _ _ _ _ _]
      event Timeout {
        n250 = event-data() -> ()  [unwired: 1 in, 3 out]
      }
      event "Display Browser Back to main menu": Value Change {
        n251 = event-data() -> ()  [unwired: 1 in, 6 out]
        n252 = property on="Tab Control" class="TabCtl (strict)"("Val(Sgnl)"=T1."Main Menu" ("Value (Signaling)")) -> ()  [unwired: 2 in, 2 out]
      }
      event "Door control Back to Main Menu": Value Change {
        n253 = event-data() -> ()  [unwired: 1 in, 6 out]
        n254 = property on="Tab Control" class="TabCtl (strict)"("Val(Sgnl)"=T1."Main Menu" ("Value (Signaling)")) -> ()  [unwired: 2 in, 2 out]
      }
      event "Inner Control Back to Main Menu": Value Change {
        n255 = event-data() -> ()  [unwired: 1 in, 6 out]
        n256 = property on="Tab Control" class="TabCtl (strict)"("Val(Sgnl)"=T1."Main Menu" ("Value (Signaling)")) -> ()  [unwired: 2 in, 2 out]
      }
      event "Radio Back to main menu": Value Change {
        n257 = event-data() -> ()  [unwired: 1 in, 6 out]
        n258 = property on="Tab Control" class="TabCtl (strict)"("Val(Sgnl)"=T1."Main Menu" ("Value (Signaling)")) -> ()  [unwired: 2 in, 2 out]
      }
      event "Browser Back to Main Menu": Value Change {
        n259 = event-data() -> ()  [unwired: 1 in, 6 out]
        n260 = property on="Tab Control" class="TabCtl (strict)"("Val(Sgnl)"=T1."Main Menu" ("Value (Signaling)")) -> ()  [unwired: 2 in, 2 out]
      }
      event "Outer Control Back to Main Menu": Value Change {
        n261 = event-data() -> ()  [unwired: 1 in, 6 out]
        n262 = property on="Tab Control" class="TabCtl (strict)"("Val(Sgnl)"=T1."Main Menu" ("Value (Signaling)")) -> ()  [unwired: 2 in, 2 out]
      }
      event "Main Menu Log Out": Value Change {
        n263 = event-data() -> ()  [unwired: 1 in, 6 out]
        n264 = property on="Tab Control" class="TabCtl (strict)"("Val(Sgnl)"=T1."Login Page" ("Value (Signaling)")) -> ()  [unwired: 2 in, 2 out]
      }
    }
  }
  n265 = while {
    tunnel: w31 -> [w293]
    tunnel: [w292] -> w30
    stop <- w291 stop-if-true
    n266 = event shown="[14] \"Right Front Window\": Value Change" {
      selector: _ -> [_ _ _ _ _ _ _ _ _ _ _ _ _ _ _ _ _ _ _ _]
      dyn-events: _ -> [_ _ _ _ _ _ _ _ _ _ _ _ _ _ _ _ _ _ _ _]
      timeout: _ -> [_ _ _ _ _ _ _ _ _ _ _ _ _ _ _ _ _ _ _ _]
      tunnel: [_ w300 w304 w310 w314 w318 w322 w326 w330 w334 w338 w342 w347 w351 w355 w359 w363 w367 w371 w375] -> w290
      tunnel: [TRUE _ _ _ _ _ _ _ _ _ _ _ _ _ _ _ _ _ _ _] -> w291
      event Timeout {
        n267 = event-data() -> ()  [unwired: 1 in, 3 out]
      }
      event "Low Light Beam": Value Change {
        n268 = event-data() -> ()  [unwired: 1 in, 6 out]
        n269 = Type Cast(x="Low Light Beam") -> (*(type *) &x=w301:string)  [unwired: 1 in]
        n270 = Concatenate Strings "Concatenate Strings"("01" ("string"), w301) -> (w300:string)
      }
      event "Close All Windows": Value Change {
        n271 = event-data() -> ()  [unwired: 1 in, 6 out]
        n272 = Type Cast(x="Close All Windows") -> (*(type *) &x=w305:string)  [unwired: 1 in]
        n273 = case shown="False" "Close All Windows" {
          frame True {
            w306 = 100
            n274 = local write "Left Back Window"(w306) -> ()
            n275 = local write "Right Front Window"(w306) -> ()
            n276 = local write "Right Back Window"(w306) -> ()
            n277 = local write "Left Front Window"(w306) -> ()
          }
          frame False {
            w307 = 0
            n278 = local write "Left Back Window"(w307) -> ()
            n279 = local write "Right Front Window"(w307) -> ()
            n280 = local write "Right Back Window"(w307) -> ()
            n281 = local write "Left Front Window"(w307) -> ()
          }
        }
        n282 = Concatenate Strings "Concatenate Strings"("02" ("string"), w305) -> (w304:string)
      }
      event "Window  Child Lock": Value Change {
        n283 = event-data() -> ()  [unwired: 1 in, 6 out]
        n284 = Type Cast(x="Window  Child Lock") -> (*(type *) &x=w311:string)  [unwired: 1 in]
        n285 = Concatenate Strings "Concatenate Strings"("03" ("string"), w311) -> (w310:string)
      }
      event "Close Moonroof": Value Change {
        n286 = event-data() -> ()  [unwired: 1 in, 6 out]
        n287 = Type Cast(x="Close Moonroof") -> (*(type *) &x=w315:string)  [unwired: 1 in]
        n288 = Concatenate Strings "Concatenate Strings"("04" ("string"), w315) -> (w314:string)
      }
      event "High Light Beam": Value Change {
        n289 = event-data() -> ()  [unwired: 1 in, 6 out]
        n290 = Type Cast(x="High Light Beam") -> (*(type *) &x=w319:string)  [unwired: 1 in]
        n291 = Concatenate Strings "Concatenate Strings"("06" ("string"), w319) -> (w318:string)
      }
      event "Front Right Door": Value Change {
        n292 = event-data() -> ()  [unwired: 1 in, 6 out]
        n293 = Type Cast(x="Front Right Door") -> (*(type *) &x=w323:string)  [unwired: 1 in]
        n294 = Concatenate Strings "Concatenate Strings"("07" ("string"), w323) -> (w322:string)
      }
      event "Back Right Door": Value Change {
        n295 = event-data() -> ()  [unwired: 1 in, 6 out]
        n296 = Type Cast(x="Back Right Door") -> (*(type *) &x=w327:string)  [unwired: 1 in]
        n297 = Concatenate Strings "Concatenate Strings"("08" ("string"), w327) -> (w326:string)
      }
      event "Front Left Door": Value Change {
        n298 = event-data() -> ()  [unwired: 1 in, 6 out]
        n299 = Type Cast(x="Front Left Door") -> (*(type *) &x=w331:string)  [unwired: 1 in]
        n300 = Concatenate Strings "Concatenate Strings"("09" ("string"), w331) -> (w330:string)
      }
      event "Back Left Door": Value Change {
        n301 = event-data() -> ()  [unwired: 1 in, 6 out]
        n302 = Type Cast(x="Back Left Door") -> (*(type *) &x=w335:string)  [unwired: 1 in]
        n303 = Concatenate Strings "Concatenate Strings"("10" ("string"), w335) -> (w334:string)
      }
      event "Lock All Doors": Value Change {
        n304 = event-data() -> ()  [unwired: 1 in, 6 out]
        n305 = Type Cast(x="Lock All Doors") -> (*(type *) &x=w339:string)  [unwired: 1 in]
        n306 = Concatenate Strings "Concatenate Strings"("11" ("string"), w339) -> (w338:string)
      }
      event "Close All Doors": Value Change {
        n307 = event-data() -> ()  [unwired: 1 in, 6 out]
        n308 = Type Cast(x="Close All Doors") -> (*(type *) &x=w343:string)  [unwired: 1 in]
        n309 = Concatenate Strings "Concatenate Strings"("12" ("string"), w343) -> (w342:string)
      }
      event "Left Front Window": Value Change {
        n310 = event-data() -> ()  [unwired: 1 in, 6 out]
        n311 = Number To Decimal String(number="Left Front Window") -> (decimal integer string=w344:string)  [unwired: 1 in]
        n312 = Concatenate Strings "Concatenate Strings"("14" ("string"), w344) -> (w347:string)
      }
      event "Left Back Window": Value Change {
        n313 = event-data() -> ()  [unwired: 1 in, 6 out]
        n314 = Number To Decimal String(number="Left Back Window") -> (decimal integer string=w349:string)  [unwired: 1 in]
        n315 = Concatenate Strings "Concatenate Strings"("15" ("string"), w349) -> (w351:string)
      }
      event "Right Front Window": Value Change {
        n316 = event-data() -> ()  [unwired: 1 in, 6 out]
        n317 = Number To Decimal String(number="Right Front Window") -> (decimal integer string=w353:string)  [unwired: 1 in]
        n318 = Concatenate Strings "Concatenate Strings"("16" ("string"), w353) -> (w355:string)
      }
      event "Right Back Window": Value Change {
        n319 = event-data() -> ()  [unwired: 1 in, 6 out]
        n320 = Number To Decimal String(number="Right Back Window") -> (decimal integer string=w357:string)  [unwired: 1 in]
        n321 = Concatenate Strings "Concatenate Strings"("17" ("string"), w357) -> (w359:string)
      }
      event "Trunk 2": Value Change {
        n322 = event-data() -> ()  [unwired: 1 in, 6 out]
        n323 = Type Cast(x="Trunk 2") -> (*(type *) &x=w361:string)  [unwired: 1 in]
        n324 = Concatenate Strings "Concatenate Strings"("18" ("string"), w361) -> (w363:string)
      }
      event "Bonnet 2": Value Change {
        n325 = event-data() -> ()  [unwired: 1 in, 6 out]
        n326 = Type Cast(x="Bonnet 2") -> (*(type *) &x=w365:string)  [unwired: 1 in]
        n327 = Concatenate Strings "Concatenate Strings"("19" ("string"), w365) -> (w367:string)
      }
      event "Oil Tank": Value Change {
        n328 = event-data() -> ()  [unwired: 1 in, 6 out]
        n329 = Type Cast(x="Oil Tank") -> (*(type *) &x=w369:string)  [unwired: 1 in]
        n330 = Concatenate Strings "Concatenate Strings"("21" ("string"), w369) -> (w371:string)
      }
      event "Double Signal": Value Change {
        n331 = event-data() -> ()  [unwired: 1 in, 6 out]
        n332 = Type Cast(x="Double Signal") -> (*(type *) &x=w373:string)  [unwired: 1 in]
        n333 = Concatenate Strings "Concatenate Strings"("20" ("string"), w373) -> (w375:string)
      }
    }
    n334 = String Length(string=w290) -> (length=w295:i32)
    n335 = Type Cast(x=w295) -> (*(type *) &x=w296:string)  [unwired: 1 in]
    n336 = TCP Write(connection ID=w293, data in=w296) -> (error out=w294:errorcluster)  [unwired: 2 in, 2 out]
    n337 = TCP Write(connection ID=w293, data in=w290, error in (no error)=w294) -> (connection ID out=w292:refnum<k5>)  [unwired: 1 in, 2 out]
  }
  n338 = while {
    stop <- FALSE stop-if-true
    n339 = local read "Lock All Doors"() -> (w377:bool)
    n340 = case shown="False" w377 {
      frame True {
        n341 = property on="Front Right Door" class="Bool (strict)"("DisabledEnum"=T5."Disabled and Grayed Out" ("Disabled")) -> ()  [unwired: 2 in, 2 out]
        n342 = property on="Back Right Door" class="Bool (strict)"("DisabledEnum"=T5."Disabled and Grayed Out" ("Disabled")) -> ()  [unwired: 2 in, 2 out]
        n343 = property on="Front Left Door" class="Bool (strict)"("DisabledEnum"=T5."Disabled and Grayed Out" ("Disabled")) -> ()  [unwired: 2 in, 2 out]
        n344 = property on="Close All Doors" class="Bool (strict)"("DisabledEnum"=T5."Disabled and Grayed Out" ("Disabled")) -> ()  [unwired: 2 in, 2 out]
        n345 = property on="Back Left Door" class="Bool (strict)"("DisabledEnum"=T5."Disabled and Grayed Out" ("Disabled")) -> ()  [unwired: 2 in, 2 out]
      }
      frame False {
        n346 = property on="Front Right Door" class="Bool (strict)"("DisabledEnum"=T5."Enabled" ("Disabled")) -> ()  [unwired: 2 in, 2 out]
        n347 = property on="Back Right Door" class="Bool (strict)"("DisabledEnum"=T5."Enabled" ("Disabled")) -> ()  [unwired: 2 in, 2 out]
        n348 = property on="Front Left Door" class="Bool (strict)"("DisabledEnum"=T5."Enabled" ("Disabled")) -> ()  [unwired: 2 in, 2 out]
        n349 = property on="Close All Doors" class="Bool (strict)"("DisabledEnum"=T5."Enabled" ("Disabled")) -> ()  [unwired: 2 in, 2 out]
        n350 = property on="Back Left Door" class="Bool (strict)"("DisabledEnum"=T5."Enabled" ("Disabled")) -> ()  [unwired: 2 in, 2 out]
      }
    }
  }
  n351 = while {
    stop <- FALSE stop-if-true
    n352 = event shown="[5] \"Search Button\": Value Change" {
      selector: _ -> [_ _ _ _ _ _]
      dyn-events: _ -> [_ _ _ _ _ _]
      timeout: _ -> [_ _ _ _ _ _]
      tunnel: "WebBrowser" -> [w395 w401 w407 w413 w419 w425]
      event "Google Button": Value Change {
        w393 = "http://www.google.com"  # urlString
        n353 = event-data() -> ()  [unwired: 1 in, 6 out]
        n354 = invoke on="Invoke Node" class="WebBrowser" method="Navigate"(reference=w395, "urlString"=w393) -> (reference out=w394:refnum<k24>, error out=w392:errorcluster)  [unwired: 2 in, 2 out]
        n355 = property on="Tab Control" class="TabCtl (strict)"("Val(Sgnl)"=T1."Display Browser" ("Value (Signaling)")) -> ()  [unwired: 2 in, 2 out]
        n356 = call <vilib>:"Clear Errors.vi"("error in (no error)"=w392) -> ("error out"=w391:errorcluster)  [unwired: 5 in, 1 out]
        n357 = Close Reference(reference=w394, error in (no error)=w391) -> ()  [unwired: 1 out]
      }
      event "Miscrsoft button": Value Change {
        w399 = "https://www.microsoft.com/en-my"  # urlString
        n358 = event-data() -> ()  [unwired: 1 in, 6 out]
        n359 = invoke on="Invoke Node" class="WebBrowser" method="Navigate"(reference=w401, "urlString"=w399) -> (reference out=w400:refnum<k24>, error out=w398:errorcluster)  [unwired: 2 in, 2 out]
        n360 = property on="Tab Control" class="TabCtl (strict)"("Val(Sgnl)"=T1."Display Browser" ("Value (Signaling)")) -> ()  [unwired: 2 in, 2 out]
        n361 = call <vilib>:"Clear Errors.vi"("error in (no error)"=w398) -> ("error out"=w397:errorcluster)  [unwired: 5 in, 1 out]
        n362 = Close Reference(reference=w400, error in (no error)=w397) -> ()  [unwired: 1 out]
      }
      event "Gmail button": Value Change {
        w405 = "https://mail.google.com/mail/u/0/#inbox"  # urlString
        n363 = event-data() -> ()  [unwired: 1 in, 6 out]
        n364 = invoke on="Invoke Node" class="WebBrowser" method="Navigate"(reference=w407, "urlString"=w405) -> (reference out=w406:refnum<k24>, error out=w404:errorcluster)  [unwired: 2 in, 2 out]
        n365 = property on="Tab Control" class="TabCtl (strict)"("Val(Sgnl)"=T1."Display Browser" ("Value (Signaling)")) -> ()  [unwired: 2 in, 2 out]
        n366 = call <vilib>:"Clear Errors.vi"("error in (no error)"=w404) -> ("error out"=w403:errorcluster)  [unwired: 5 in, 1 out]
        n367 = Close Reference(reference=w406, error in (no error)=w403) -> ()  [unwired: 1 out]
      }
      event "Facebook button": Value Change {
        w411 = "https://www.facebook.com/login/"  # urlString
        n368 = event-data() -> ()  [unwired: 1 in, 6 out]
        n369 = invoke on="Invoke Node" class="WebBrowser" method="Navigate"(reference=w413, "urlString"=w411) -> (reference out=w412:refnum<k24>, error out=w410:errorcluster)  [unwired: 2 in, 2 out]
        n370 = property on="Tab Control" class="TabCtl (strict)"("Val(Sgnl)"=T1."Display Browser" ("Value (Signaling)")) -> ()  [unwired: 2 in, 2 out]
        n371 = call <vilib>:"Clear Errors.vi"("error in (no error)"=w410) -> ("error out"=w409:errorcluster)  [unwired: 5 in, 1 out]
        n372 = Close Reference(reference=w412, error in (no error)=w409) -> ()  [unwired: 1 out]
      }
      event "Netflix Button": Value Change {
        w417 = "https://www.netflix.com/my-en/"  # urlString
        n373 = event-data() -> ()  [unwired: 1 in, 6 out]
        n374 = invoke on="Invoke Node" class="WebBrowser" method="Navigate"(reference=w419, "urlString"=w417) -> (reference out=w418:refnum<k24>, error out=w416:errorcluster)  [unwired: 2 in, 2 out]
        n375 = property on="Tab Control" class="TabCtl (strict)"("Val(Sgnl)"=T1."Display Browser" ("Value (Signaling)")) -> ()  [unwired: 2 in, 2 out]
        n376 = call <vilib>:"Clear Errors.vi"("error in (no error)"=w416) -> ("error out"=w415:errorcluster)  [unwired: 5 in, 1 out]
        n377 = Close Reference(reference=w418, error in (no error)=w415) -> ()  [unwired: 1 out]
      }
      event "Search Button": Value Change {
        n378 = event-data() -> ()  [unwired: 1 in, 6 out]
        n379 = invoke on="Invoke Node" class="WebBrowser" method="Navigate"(reference=w425, "urlString"="Enter Url") -> (reference out=w424:refnum<k24>, error out=w422:errorcluster)  [unwired: 2 in, 2 out]
        n380 = property on="Tab Control" class="TabCtl (strict)"("Val(Sgnl)"=T1."Display Browser" ("Value (Signaling)")) -> ()  [unwired: 2 in, 2 out]
        n381 = call <vilib>:"Clear Errors.vi"("error in (no error)"=w422) -> ("error out"=w421:errorcluster)  [unwired: 5 in, 1 out]
        n382 = Close Reference(reference=w424, error in (no error)=w421) -> ()  [unwired: 1 out]
      }
    }
  }
  n383 = local write "On/Off fan"(FALSE ("On/Off fan")) -> ()
  n384 = local read "WindowsMediaPlayer"() -> (w9:refnum<k7>)
  n385 = local write "fan light"(FALSE ("Air Conditional light")) -> ()
  n386 = Automation Open(Automation Refnum=w9) -> (Automation Refnum=w8:refnum<k7>)  [unwired: 3 in, 1 out]
  n387 = local write "On/Off Ac"(FALSE ("Ac button")) -> ()
  n388 = invoke class="IWMPPlayer4" method="close"(reference=w8) -> (reference out=w7:refnum<k7>)  [unwired: 2 in, 2 out]
  n389 = while {
    stop <- FALSE stop-if-true
    n390 = event shown="[3] \"Inner Control\": Value Change" {
      selector: _ -> [_ _ _ _ _ _]
      dyn-events: _ -> [_ _ _ _ _ _]
      timeout: _ -> [_ _ _ _ _ _]
      event Timeout {
        n391 = event-data() -> ()  [unwired: 1 in, 3 out]
      }
      event "Door Control": Value Change {
        n392 = event-data() -> ()  [unwired: 1 in, 6 out]
        n393 = property on="Tab Control" class="TabCtl (strict)"("Val(Sgnl)"=T1."Door Control" ("Value (Signaling)")) -> ()  [unwired: 2 in, 2 out]
      }
      event "Outer Control": Value Change {
        n394 = event-data() -> ()  [unwired: 1 in, 6 out]
        n395 = property on="Tab Control" class="TabCtl (strict)"("Val(Sgnl)"=T1."Outer Control" ("Value (Signaling)")) -> ()  [unwired: 2 in, 2 out]
      }
      event "Inner Control": Value Change {
        n396 = event-data() -> ()  [unwired: 1 in, 6 out]
        n397 = property on="Tab Control" class="TabCtl (strict)"("Val(Sgnl)"=T1."Inner Control" ("Value (Signaling)")) -> ()  [unwired: 2 in, 2 out]
      }
      event "Radio": Value Change {
        n398 = event-data() -> ()  [unwired: 1 in, 6 out]
        n399 = property on="Tab Control" class="TabCtl (strict)"("Val(Sgnl)"=T1."Radio" ("Value (Signaling)")) -> ()  [unwired: 2 in, 2 out]
      }
      event "Broswer": Value Change {
        n400 = event-data() -> ()  [unwired: 1 in, 6 out]
        n401 = property on="Tab Control" class="TabCtl (strict)"("Val(Sgnl)"=T1."Browser" ("Value (Signaling)")) -> ()  [unwired: 2 in, 2 out]
      }
    }
  }
  n402 = Get Date/Time In Seconds() -> (seconds since 1Jan1904=→"current time 4":timestamp)
  n403 = Get Date/Time In Seconds() -> (seconds since 1Jan1904=→"current time 24":timestamp)
  n404 = Get Date/Time In Seconds() -> (seconds since 1Jan1904=→"current time 6":timestamp)
  n405 = Get Date/Time In Seconds() -> (seconds since 1Jan1904=→"current time 8":timestamp)
  n406 = Get Date/Time In Seconds() -> (seconds since 1Jan1904=→"current time 16":timestamp)
  n407 = Get Date/Time In Seconds() -> (seconds since 1Jan1904=→"current time 10":timestamp)
  n408 = Get Date/Time In Seconds() -> (seconds since 1Jan1904=→"current time 12":timestamp)
  n409 = Get Date/Time In Seconds() -> (seconds since 1Jan1904=→"current time 22":timestamp)
  n410 = Get Date/Time In Seconds() -> (seconds since 1Jan1904=→"current time 2":timestamp)
  n411 = TCP Close Connection(connection ID=w30) -> ()  [unwired: 2 in, 2 out]
  n412 = local write "Ac light"(FALSE ("Ac light")) -> ()
  n413 = Close Reference(reference=w7) -> ()  [unwired: 1 in, 1 out]
  "Display channel" <- "" ("String")
  "Boolean 2" <- FALSE ("Boolean 2")
